vi "Graphics-Draw X (Picture).vi"(0 "picture in":picture, 7 "rect":T1, 12 "color(black)":u32(colorbox)=16711680, 13 "pen":T2) -> (4 "picture out":picture)   [LabVIEW 2020]
uses:
  <vilib>/Utility/miscctls.llb/LVRectTypeDef.ctl
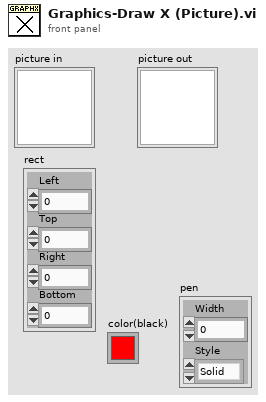
[diagram p1: front panel]
types:
  T1 = typedef "LVRectTypeDef.ctl" = cluster{"Left":i16, "Top":i16, "Right":i16, "Bottom":i16}
  T2 = cluster{"Width":u16, "Style":enum32{"Solid", "Dash", "Dot", "DashDot", "DashDotDot"}}
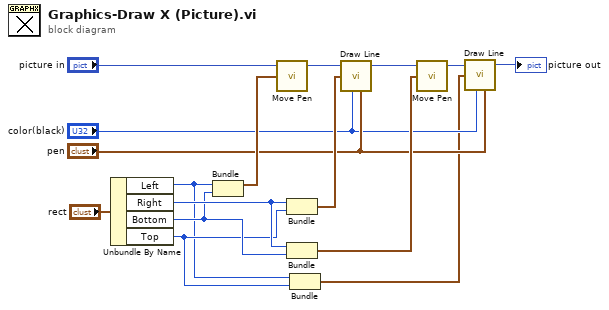
[diagram p0: block diagram]
diagram:
  n1 = Unbundle By Name("rect") -> ("Left"=w2:i16, "Right"=w10:i16, "Bottom"=w9:i16, "Top"=w3:i16)
  n2 = Bundle("Left"=w2, "Bottom"=w9) -> (w13:cluster{"Left":i16, "Bottom":i16})  [unwired: 1 in]
  n3 = call <vilib>:"Move Pen.vi"("new position"=w13, "picture"="picture in") -> ("new picture"=w14:picture)  [unwired: 3 in]
  n4 = Bundle("Right"=w10, "Top"=w3) -> (w12:cluster{"Right":i16, "Top":i16})  [unwired: 1 in]
  n5 = Bundle("Right"=w10, "Bottom"=w9) -> (w8:cluster{"Right":i16, "Bottom":i16})  [unwired: 1 in]
  n6 = Bundle("Left"=w2, "Top"=w3) -> (w1:cluster{"Left":i16, "Top":i16})  [unwired: 1 in]
  n7 = call <vilib>:"Draw Line.vi"("picture"=w14, "end point"=w12, "color(black)"="color(black)", "pen"="pen") -> ("new picture"=w11:picture)  [unwired: 5 in]
  n8 = call <vilib>:"Move Pen.vi"("new position"=w8, "picture"=w11) -> ("new picture"=w7:picture)  [unwired: 3 in]
  n9 = call <vilib>:"Draw Line.vi"("picture"=w7, "end point"=w1, "color(black)"="color(black)", "pen"="pen") -> ("new picture"=→"picture out":picture)  [unwired: 5 in]
